vi "BK Precision 8500 Control Panel.vi"() -> ()   [LabVIEW 2010]
doc: "This example VI demonstrates how to setup the instrument to sink a desired current at the input terminal."
uses:
  <instrlib>/BK Precision 85XX Series/BK Precision 85XX Series.lvlib
panel:
  in  "?":bool
  out "Requested\nVoltage":dbl
  in  "stop":bool
  out "Voltage":dbl
  out "Power":dbl
  out "Current":dbl
  in  "COM Port":refnum<visa-resource-name>
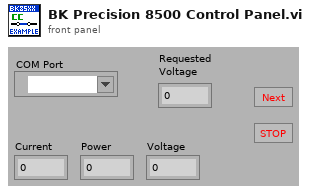
[diagram p1: front panel]
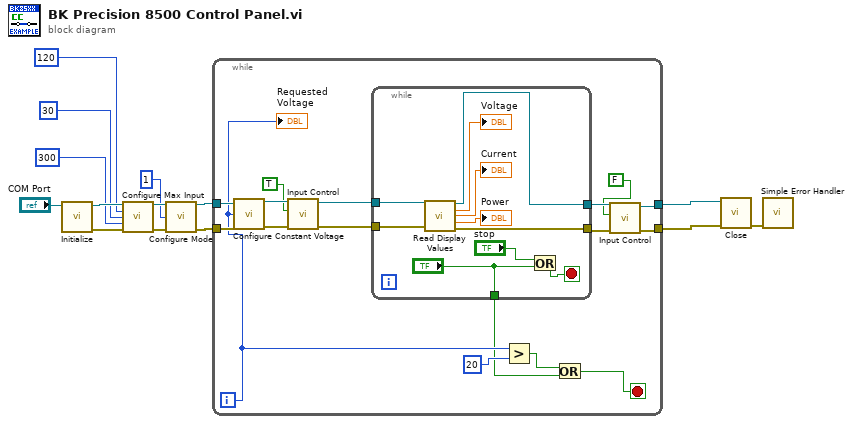
[diagram p0: block diagram]
diagram:
  n1 = call <instrlib>:"Initialize.vi"("VISA resource name"="COM Port") -> ("error out"=w12:errorcluster, "VISA resource name out"=w13:refnum<visa-resource-name>)  [unwired: 9 in]
  n2 = call <instrlib>:"Configure Max Input.vi"("VISA resource name"=w13, "Maximum Input Voltage (0)"=120, "Maximum Input Current (0)"=30, "Maximum Input Power (0)"=300, "error in (no error)"=w12) -> ("VISA resource name out"=w11:refnum<visa-resource-name>, "error out"=w10:errorcluster)  [unwired: 9 in]
  n3 = call <instrlib>:"Configure Mode.vi"("VISA resource name"=w11, "Mode of Operation (0:CC)"=1, "error in (no error)"=w10) -> ("VISA resource name out"=w5:refnum<visa-resource-name>, "error out"=w4:errorcluster)  [unwired: 11 in]
  n4 = while {
    tunnel: [w22] -> w8
    tunnel: [w20] -> w7
    tunnel: w5 -> [w31]
    tunnel: w4 -> [w30]
    i -> [w18]
    stop <- w17 stop-if-true
    n5 = call <instrlib>:"Configure Constant Voltage.vi"("VISA resource name"=w31, "CV Voltage (0)"=w18, "error in (no error)"=w30) -> ("VISA resource name out"=w28:refnum<visa-resource-name>, "error out"=w27:errorcluster)  [unwired: 11 in]
    n6 = call <instrlib>:"Input Control.vi"("error in (no error)"=w27, "Enable Input Terminals (F: Off)"=TRUE, "VISA resource name"=w28) -> ("error out"=w24:errorcluster, "VISA resource name out"=w25:refnum<visa-resource-name>)  [unwired: 7 in]
    n7 = while {
      tunnel: [w41] -> w21
      tunnel: [w40] -> w23
      tunnel: w25 -> [w36]
      tunnel: w24 -> [w35]
      tunnel: ["?"] -> w15
      stop <- w33 stop-if-true
      n8 = call <instrlib>:"Read Display Values.vi"("VISA resource name"=w36, "error in (no error)"=w35) -> ("VISA resource name out"=w40:refnum<visa-resource-name>, "Terminal Input Voltage (V)"=→"Voltage":dbl, "Terminal Input Current (A)"=→"Current":dbl, "Terminal Input Power (W)"=→"Power":dbl, "error out"=w41:errorcluster)  [unwired: 9 in]
      n9 = Or(x="stop", y="?") -> (x .or. y?=w33:bool)
    }
    n10 = Greater?(x=w18, y=20) -> (0:w16:bool)
    n11 = Or(x=w16, y=w15) -> (x .or. y?=w17:bool)
    n12 = call <instrlib>:"Input Control.vi"("error in (no error)"=w21, "Enable Input Terminals (F: Off)"=FALSE, "VISA resource name"=w23) -> ("error out"=w20:errorcluster, "VISA resource name out"=w22:refnum<visa-resource-name>)  [unwired: 7 in]
    "Requested\nVoltage" <- w18
  }
  n13 = call <instrlib>:"Close.vi"("error in (no error)"=w7, "VISA resource name"=w8) -> ("error out"=w9:errorcluster)  [unwired: 9 in]
  n14 = call <vilib>:"Simple Error Handler.vi"("error in (no error)"=w9) -> ()  [unwired: 4 in, 5 out]
